vi "Ex4_DataTypes.vi"() -> ()   [LabVIEW 2024]
panel:
  out "Indicator 4":string
  out "Indicator 2":i32
  out "Indicator 1":dbl
  out "Indicator 3":bool
  in  "Input 2":i32
  in  "Input 1":dbl
  in  "Input 4":string
  in  "Input 3":bool
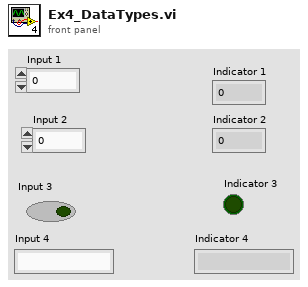
[diagram p1: front panel]
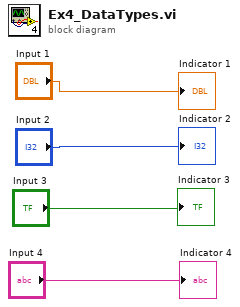
[diagram p0: block diagram]
diagram:
  "Indicator 3" <- "Input 3"
  "Indicator 1" <- "Input 1"
  "Indicator 2" <- "Input 2"
  "Indicator 4" <- "Input 4"
